vi "handle_data.vi"(0 "串口数据":string) -> (1 "数据文件路径":path, 2 "解析数据":string[][](array[string]))   [LabVIEW 2018]
panel:
  out "卡位":string
  out "槽位":string
  out "测量板卡":u32[][](array[colorbox])
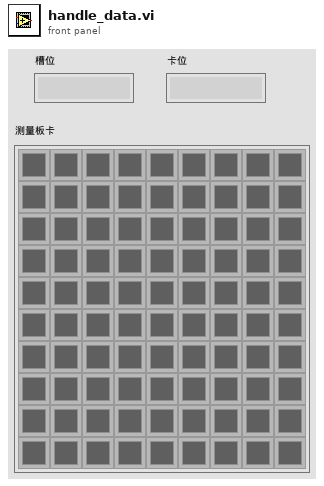
[diagram p1: front panel]
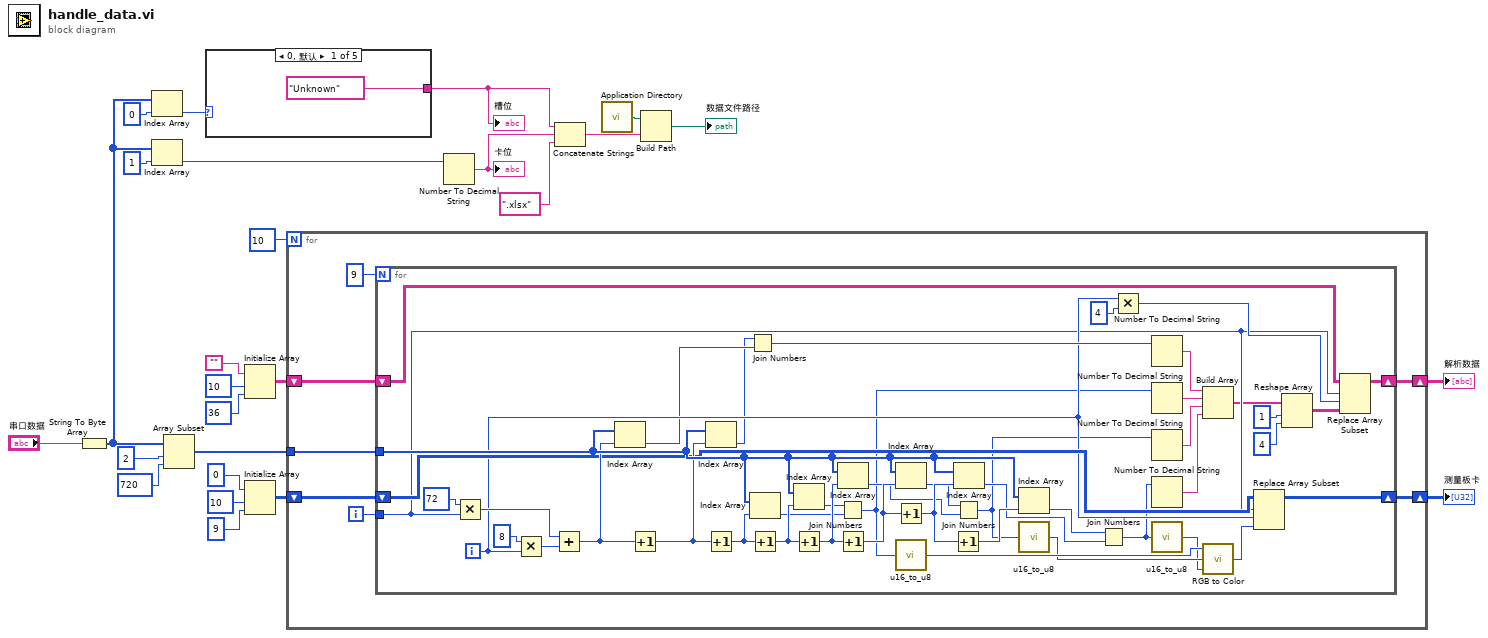
[diagram p0: block diagram]
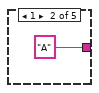
[diagram p2: hidden frame]
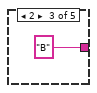
[diagram p3: hidden frame]
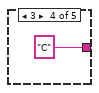
[diagram p4: hidden frame]
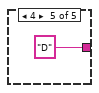
[diagram p5: hidden frame]
diagram:
  n1 = String To Byte Array(string="串口数据") -> (unsigned byte array=w4:u8[])
  n2 = Index Array(array=w4, index=0 ("索引")) -> (element=w24:u8)
  n3 = Index Array(array=w4, index=1 ("索引")) -> (element=w21:u8)
  n4 = Array Subset(array=w4, index=2 ("索引"), length=720 ("长度")) -> (w5:u8[])
  n5 = case shown="0, 默认" w24 {
    tunnel: ["Unknown" "A" "B" "C" "D"] -> w23
    frame 0, Default {
    }
    frame 1 {
    }
    frame 2 {
    }
    frame 3 {
    }
    frame 4 {
    }
  }
  "槽位" <- w23
  n6 = Initialize Array("", 10 ("维数大小"), 36 ("维数大小")) -> (w8:string[][])
  n7 = Initialize Array(u32 0, 10 ("维数大小"), 9 ("维数大小")) -> (w13:u32[][])
  n8 = for {
    N: 10 -> [_]
    tunnel: w5 -> [w37]
    shift-right: [w34] -> w12
    shift-left: w13 -> [w35]
    shift-right: [w32] -> w7
    shift-left: w8 -> [w33]
    i -> [w36]
    n9 = for {
      N: 9 -> [_]
      tunnel: w37 -> [w79]
      shift-right: [w63] -> w32
      shift-left: w33 -> [w65]
      tunnel: w36 -> [w43]
      shift-right: [w60] -> w34
      shift-left: w35 -> [w62]
      i -> [w61]
      n10 = Multiply(x=72, y=w43) -> (x*y=w82:i32)
      n11 = Multiply(x=8, y=w61) -> (x*y=w80:i32)
      n12 = Add(x=w82, y=w80) -> (x+y=w78:i32)
      n13 = Index Array(array=w79, index=w78) -> (element=w58:u8)
      n14 = Increment(x=w78) -> (x+1=w77:i32)
      n15 = Index Array(array=w79, index=w77) -> (element=w57:u8)
      n16 = Increment(x=w77) -> (x+1=w76:i32)
      n17 = Join Numbers(hi=w57, lo=w58) -> ((hi.lo)=w70:u16)
      n18 = Index Array(array=w79, index=w76) -> (element=w55:u8)
      n19 = Increment(x=w76) -> (x+1=w75:i32)
      n20 = Index Array(array=w79, index=w75) -> (element=w56:u8)
      n21 = Increment(x=w75) -> (x+1=w74:i32)
      n22 = Index Array(array=w79, index=w74) -> (element=w53:u8)
      n23 = Join Numbers(hi=w56, lo=w55) -> ((hi.lo)=w50:u16)
      n24 = Increment(x=w74) -> (x+1=w73:i32)
      n25 = Index Array(array=w79, index=w73) -> (element=w54:u8)
      n26 = Increment(x=w73) -> (x+1=w72:i32)
      n27 = call "u16_to_u8.vi"("数值"=w50) -> ("无符号8位整型"=w49:u8)
      n28 = Increment(x=w72) -> (x+1=w71:i32)
      n29 = Index Array(array=w79, index=w72) -> (element=w51:u8)
      n30 = Join Numbers(hi=w54, lo=w53) -> ((hi.lo)=w48:u16)
      n31 = Index Array(array=w79, index=w71) -> (element=w52:u8)
      n32 = call "u16_to_u8.vi"("数值"=w48) -> ("无符号8位整型"=w47:u8)
      n33 = Join Numbers(hi=w52, lo=w51) -> ((hi.lo)=w46:u16)
      n34 = Multiply(x=w61, y=4) -> (x*y=w44:i32)
      n35 = Number To Decimal String(number=w70) -> (decimal integer string=w69:string)  [unwired: 1 in]
      n36 = Number To Decimal String(number=w50) -> (decimal integer string=w66:string)  [unwired: 1 in]
      n37 = Number To Decimal String(number=w48) -> (decimal integer string=w68:string)  [unwired: 1 in]
      n38 = Number To Decimal String(number=w46) -> (decimal integer string=w67:string)  [unwired: 1 in]
      n39 = call "u16_to_u8.vi"("数值"=w46) -> ("无符号8位整型"=w45:u8)
      n40 = Build Array(w69, w66, w68, w67) -> (w40:string[])
      n41 = call <vilib>:"RGB to Color.vi"("B"=w45, "G"=w47, "R"=w49) -> ("Color"=w59:u32)
      n42 = Replace Array Subset(array=w62, new element=w59, index (row)=w43, index (col)=w61) -> (w60:u32[][])
      n43 = Reshape Array(w40, 1 ("维数大小"), 4 ("维数大小")) -> (w39:string[][])
      n44 = Replace Array Subset(array=w65, new element=w39, index (row)=w43, index (col)=w44) -> (w63:string[][])
    }
  }
  "测量板卡" <- w12
  "解析数据" <- w7
  n45 = Number To Decimal String(number=w21) -> (decimal integer string=w20:string)  [unwired: 1 in]
  "卡位" <- w20
  n46 = Concatenate Strings(w23, w20, ".xlsx" ("字符串")) -> (w19:string)
  n47 = call <vilib>:"Application Directory.vi"() -> ("Application Directory"=w1:path)
  n48 = Build Path(base path=w1, name or relative path=w19) -> (appended path=→"数据文件路径":path)
